vi "mydatawrite.vi"(6 "Data file name:":path=path "C:/temp/datafile_250816.lvm", 7 "File header":string="%Info. Blah. Blah.\n%Column 1: t [s]\n%Column 2: x [V]", 8 "Start_stop_file_writing":bool, 9 "SampleTime":dbl, 10 "Data2":dbl, 11 "Data1":dbl(slide) scale=0.0..10.0) -> ()   [LabVIEW 2021]
uses:
  <vilib>/Utility/file.llb/Write Delimited Spreadsheet (string).vi
panel:
  # "Start"
  # "Stop"
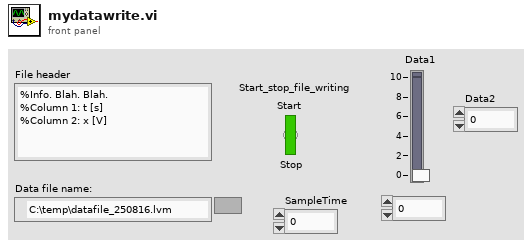
[diagram p1: front panel]
types:
  T1 = enum16{"open", "replace", "create", "open or create", "replace or create", "replace or create with confirmation"}
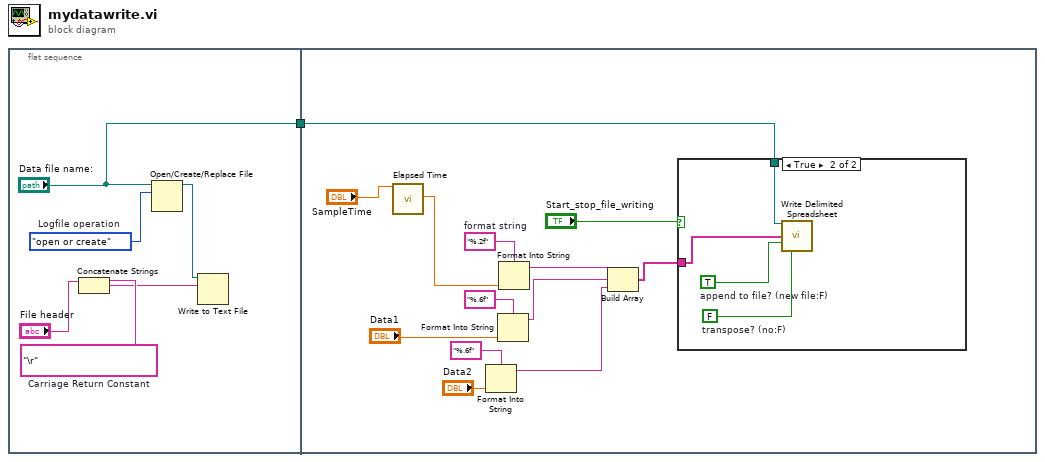
[diagram p0: block diagram]
diagram:
  n1 = flat-sequence {
    tunnel: ["Data file name:"] -> w1
    tunnel: w1 -> [w20]
    frame #0 {
      w4 = "\r"  # Carriage Return Constant
      w7 = T1."open or create"  # Logfile operation
      n2 = Concatenate Strings "Concatenate Strings"("File header", w4) -> (w2:string)
      n3 = Open/Create/Replace File(file path (use dialog)="Data file name:", operation (0:open)=w7) -> (refnum out=w6:refnum<file>)  [unwired: 4 in, 2 out]
      n4 = Write to Text File(file (use dialog)=w6, text=w2) -> ()  [unwired: 2 in, 3 out]
    }
    frame #1 {
      w17 = "%.2f"  # format string
      n5 = call "Elapsed Time"("Time Target (s)"="SampleTime") -> ("Elapsed Time (s)"=w8:dbl)  [unwired: 11 in, 7 out]
      n6 = Format Into String(format string="%.6f", "Data2") -> (resulting string=w10:string)  [unwired: 2 in, 1 out]
      n7 = Format Into String(format string="%.6f", "Data1") -> (resulting string=w14:string)  [unwired: 2 in, 1 out]
      n8 = Format Into String "Format Into String"(format string=w17, w8) -> (resulting string=w15:string)  [unwired: 2 in, 1 out]
      n9 = Build Array "Build Array"(w15, w14, w10) -> (w18:string[])
      n10 = case shown="True" "Start_stop_file_writing" {
        tunnel: w18 -> [_ w22]
        tunnel: w20 -> [_ w21]
        frame False {
        }
        frame True {
          w24 = TRUE  # append to file? (new file:F)
          w23 = FALSE  # transpose? (no:F)
          n11 = call-poly <vilib>:"Write Delimited Spreadsheet.vi"("file path (dialog if empty)"=w21, "1D data"=w22, "append to file? (new file:F)"=w24, "transpose? (no:F)"=w23) -> ()  [unwired: 10 in, 2 out]
        }
      }
    }
  }
